vi "RSZVB Format Parameter Command.vi"(8 "error in (no error)":errorcluster {"code" format="%.0x"}, 9 "Trace Name (Trc1)":string="Trc1", 10 "Channel (1)":i32=1, 11 "VISA session":refnum<visa-resource-name>) -> (0 "error out":errorcluster {"code" format="%.0x"}, 2 "Buffer":string, 3 "dup VISA session":refnum<visa-resource-name>)   [LabVIEW 2015]
doc: "This VI serves as utility VI."
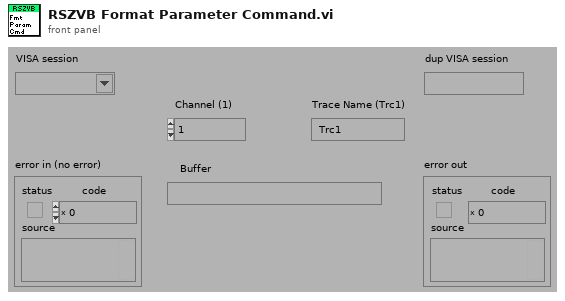
[diagram p1: front panel]
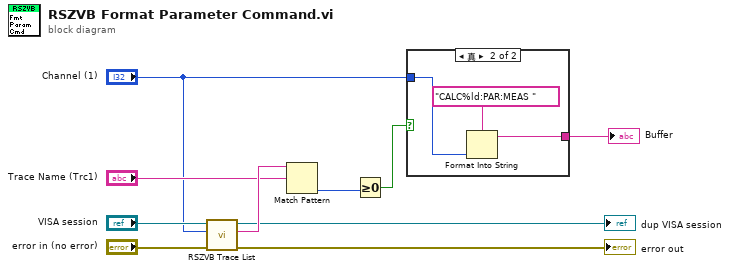
[diagram p0: block diagram]
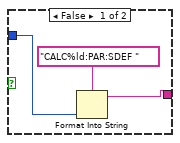
[diagram p2: hidden frame]
diagram:
  n1 = call "RSZVB Trace List.vi"("error in (no error)"="error in (no error)", "Channel (1)"="Channel (1)", "VISA session"="VISA session") -> ("error out"=→"error out":errorcluster, "Catalog"=w8:string, "dup VISA session"=→"dup VISA session":refnum<visa-resource-name>)  [unwired: 6 in]
  n2 = Match Pattern(string=w8, regular expression="Trace Name (Trc1)") -> (offset past match=w6:i32)  [unwired: 1 in, 3 out]
  n3 = Greater Or Equal To 0?(x=w6) -> (x >= 0?=w5:bool)
  n4 = case shown="真" w5 {
    tunnel: "Channel (1)" -> [w12 w15]
    tunnel: [w11 w14] -> w2
    frame False {
      n5 = Format Into String(format string="CALC%ld:PAR:SDEF ", w12) -> (resulting string=w11:string)  [unwired: 2 in, 1 out]
    }
    frame True {
      n6 = Format Into String(format string="CALC%ld:PAR:MEAS ", w15) -> (resulting string=w14:string)  [unwired: 2 in, 1 out]
    }
  }
  "Buffer" <- w2
